vi "Astar on Occupancy Grid.vi"() -> ()   [LabVIEW 2017]
doc: "This example shows how to use the A* algorithm with an occupancy grid to compute the shortest path between start and goal nodes."
uses:
  <vilib>/robotics/Navigation/shared/WorldMap/OccupancyGridWorldMap/NI_Robotics_OccupancyGridWorldMap.lvclass
panel:
  in  "Save Grid":bool
  in  "Load Grid":bool
  in  "Action":enum32{"Mark Obstacle", "Set Start", "Set Goal"}(radio)
  in  "stop":bool
  out "Intensity Graph":dbl[][](graph)
  # "This example uses the A* algorithm to compute the shortest path between a start node and a goal node on an occupancy grid.\n\n1. Click the grid with Mark Obstacle selected to add or remove obstacles in the occupancy grid.\n\n2. Click the grid with Set Start or Set Goal selected to move the start and goal nodes of the shortest path.\n\n3. Click the Save button to save the current occupancy grid to a tab delimited text file.\n\n4. Click the Load button to load an occupancy grid from a tab delimited text file."
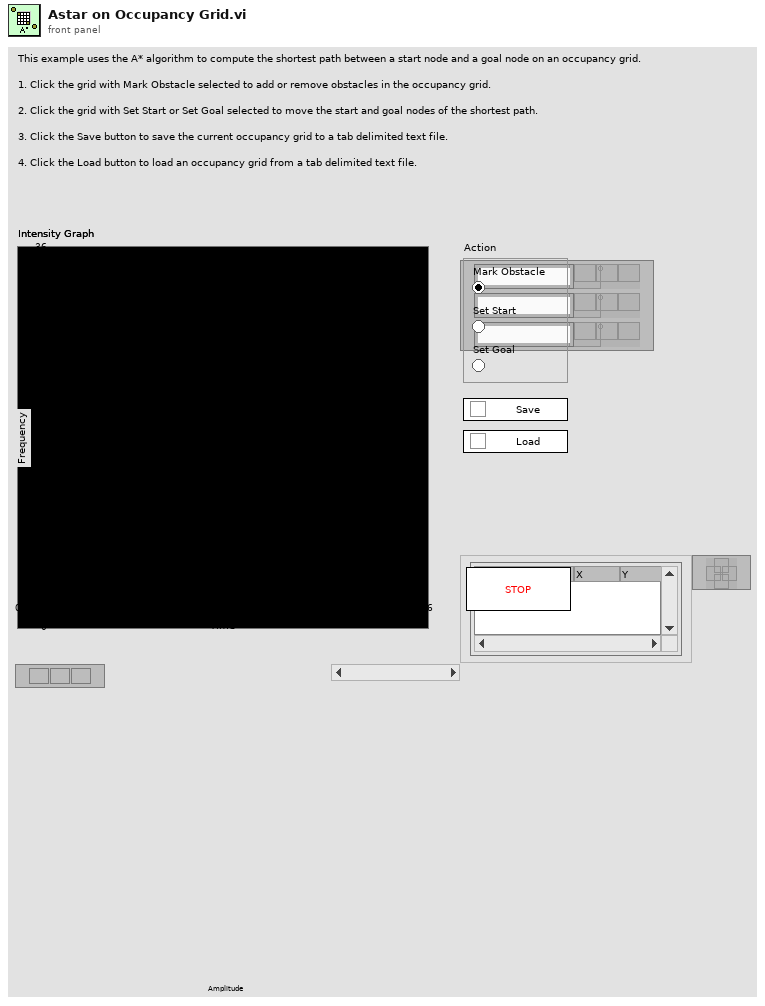
[diagram p1: front panel]
types:
  T1 = typedef "LVPoint32TypeDef.ctl" = cluster{"Horizontal":i32, "Vertical":i32}
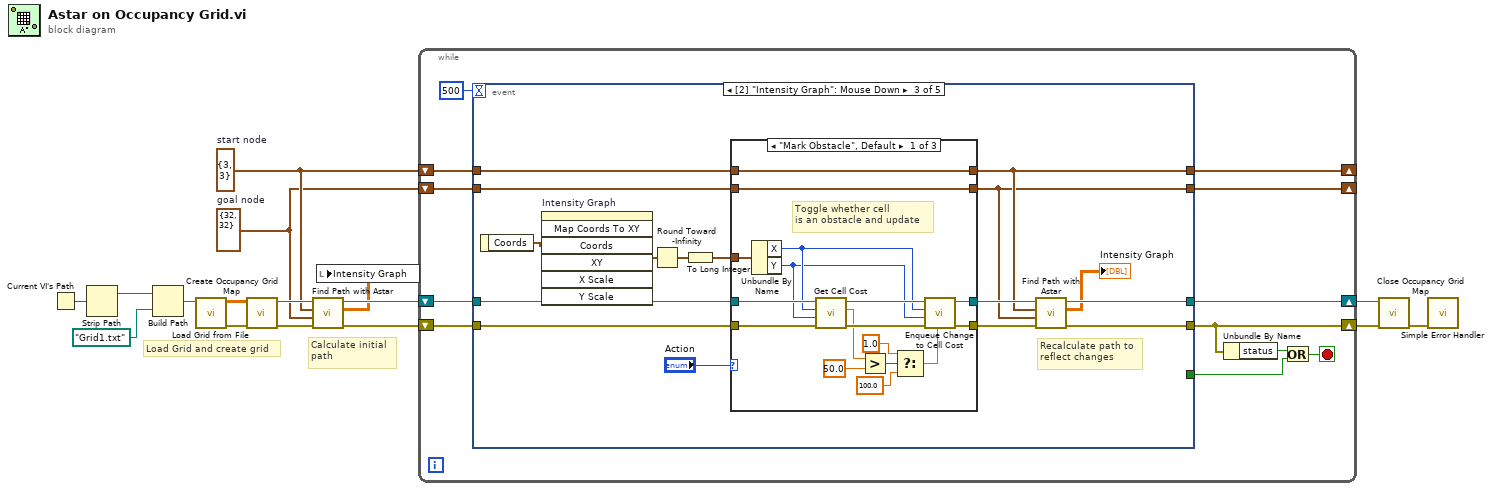
[diagram p0: block diagram]
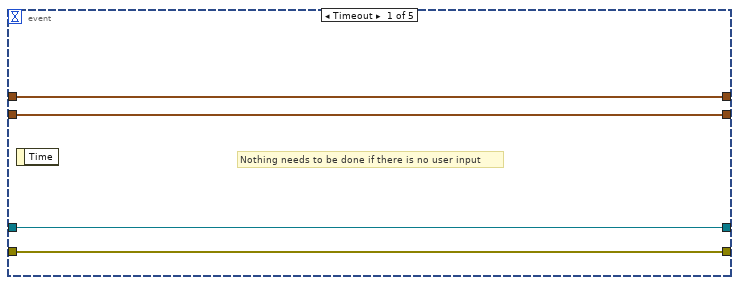
[diagram p2: hidden frame]
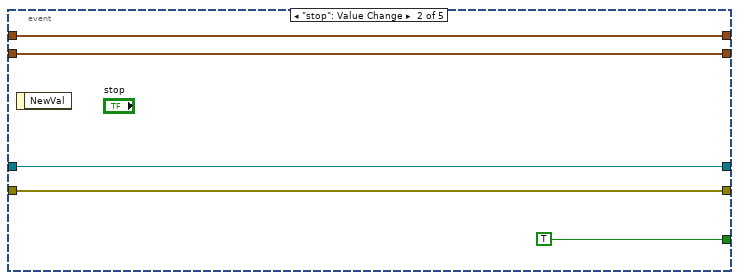
[diagram p3: hidden frame]
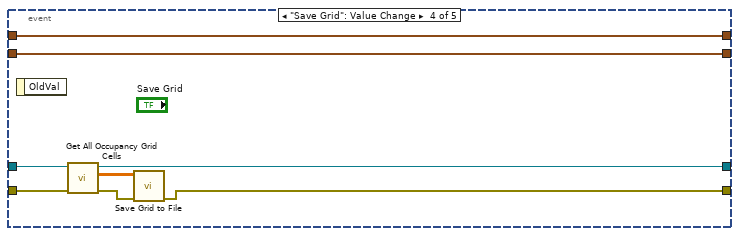
[diagram p6: hidden frame]
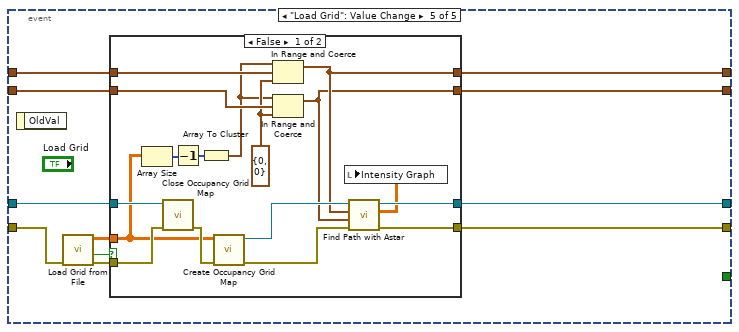
[diagram p7: hidden frame]
diagram:
  w2 = cluster{"X":i32, "Y":i32} {"X"=32, "Y"=32}  # goal node
  w3 = cluster{"X":i32, "Y":i32} {"X"=3, "Y"=3}  # start node
  # "Calculate initial \npath"
  # "Load Grid and create grid"
  n1 = Current VI's Path() -> (path=w14:path)
  n2 = Strip Path(path=w14) -> (stripped path=w13:path)  [unwired: 1 out]
  n3 = Build Path(base path=w13, name or relative path=path "Grid1.txt" ("stripped path")) -> (appended path=w11:path)
  n4 = call "Load Grid from File.vi"("file path"=w11) -> ("error out"=w9:errorcluster, "occupancy grid"=w10:dbl[][])  [unwired: 8 in, 1 out]
  n5 = call <vilib>:"Create Occupancy Grid Map.vi"("error in (no error)"=w9, "occupancy grid"=w10) -> ("error out"=w5:errorcluster, "map reference out"=w7:refnum<data-value>)  [unwired: 8 in]
  n6 = call "Find Path with Astar.vi"("error in (no error)"=w5, "goal node"=w2, "start node"=w3, "map reference in"=w7) -> ("error out"=w4:errorcluster, "intensity values"=w1:dbl[][], "map reference out"=w6:refnum<data-value>)  [unwired: 5 in]
  n7 = local write "Intensity Graph"(w1) -> ()
  n8 = while {
    shift-right: [w23] -> w16
    shift-left: w4 -> [w24]
    shift-right: [w19] -> _
    shift-left: w3 -> [w21]
    shift-right: [w18] -> _
    shift-left: w2 -> [w20]
    shift-right: [w17] -> w8
    shift-left: w6 -> [w25]
    stop <- w26 stop-if-true
    n9 = event shown="[2] \"Intensity Graph\": Mouse Down" {
      selector: _ -> [_ _ _ _ _]
      dyn-events: _ -> [_ _ _ _ _]
      timeout: 500 -> [_ _ _ _ _]
      tunnel: [_ TRUE _ _ _] -> w27
      tunnel: w25 -> [w31 w35 w50 w85 w95]
      tunnel: w24 -> [w32 w36 w49 w86 w97]
      tunnel: [w32 w36 w39 w82 w92] -> w23
      tunnel: [w31 w35 w40 w83 w91] -> w17
      tunnel: w21 -> [w30 w34 w47 w80 w90]
      tunnel: w20 -> [w29 w33 w46 w79 w89]
      tunnel: [w30 w34 w42 w80 w88] -> w19
      tunnel: [w29 w33 w41 w79 w87] -> w18
      event Timeout {
        # "Nothing needs to be done if there is no user input"
        n10 = event-data() -> ()  [unwired: 1 in, 1 out]
      }
      event "stop": Value Change {
        n11 = event-data() -> ()  [unwired: 1 in, 1 out]
      }
      event "Intensity Graph": Mouse Down {
        # "Recalculate path to\nreflect changes"
        n12 = event-data() -> ("Coords"=w53:T1)  [unwired: 1 in]
        n13 = invoke on="Intensity Graph" class="IntGraph (strict)" method="Map Coords To XY"("Coords"=w53) -> ("XY"=w52:cluster{"X":dbl, "Y":dbl})  [unwired: 6 in, 6 out]
        n14 = Round Toward -Infinity(1:w52) -> (0:w51:cluster{"X":dbl, "Y":dbl})
        n15 = To Long Integer(number=w51) -> (32bit integer=w45:cluster{"X":i32, "Y":i32})
        n16 = case shown="\"Mark Obstacle\", Default" "Action" {
          tunnel: w50 -> [w70 w72 w76]
          tunnel: w49 -> [w68 w71 w75]
          tunnel: [w60 w71 w75] -> w43
          tunnel: [w59 w72 w76] -> w44
          tunnel: w47 -> [w58 _ w78]
          tunnel: w46 -> [w57 w74 _]
          tunnel: [w58 w73 w78] -> w42
          tunnel: [w57 w74 w77] -> w41
          tunnel: w45 -> [w54 w73 w77]
          frame "Mark Obstacle", Default {
            # "Toggle whether cell\nis an obstacle and update"
            n17 = Unbundle By Name(w54) -> ("X"=w56:i32, "Y"=w55:i32)
            n18 = call <vilib>:"Get Cell Cost.vi"("error in (no error)"=w68, "y"=w55, "x"=w56, "map reference in"=w70) -> ("error out"=w67:errorcluster, "cost"=w66:dbl, "map reference out"=w69:refnum<data-value>)  [unwired: 4 in, 1 out]
            n19 = Greater?(x=w66, y=50.0) -> (0:w64:bool)
            n20 = Select(t=1.0, s=w64, f=100.0) -> (s? t:f=w61:dbl)
            n21 = call <vilib>:"Enqueue Change to Cell Cost.vi"("cost"=w61, "error in (no error)"=w67, "y"=w55, "x"=w56, "map reference in"=w69) -> ("error out"=w60:errorcluster, "map reference out"=w59:refnum<data-value>)  [unwired: 5 in]
          }
          frame "Set Start" {
            # "Change start node"
          }
          frame "Set Goal" {
            # "change goal node"
          }
        }
        n22 = call "Find Path with Astar.vi"("error in (no error)"=w43, "goal node"=w41, "start node"=w42, "map reference in"=w44) -> ("error out"=w39:errorcluster, "intensity values"=→"Intensity Graph":dbl[][], "map reference out"=w40:refnum<data-value>)  [unwired: 5 in]
      }
      event "Save Grid": Value Change {
        n23 = event-data() -> ()  [unwired: 1 in, 1 out]
        n24 = call <vilib>:"Get All Occupancy Grid Cells.vi"("error in (no error)"=w86, "map reference in"=w85) -> ("error out"=w84:errorcluster, "occupancy grid"=w81:dbl[][], "map reference out"=w83:refnum<data-value>)  [unwired: 7 in]
        n25 = call "Save Grid to File.vi"("error in (no error)"=w84, "occupancy grid"=w81) -> ("error out"=w82:errorcluster)  [unwired: 9 in]
      }
      event "Load Grid": Value Change {
        n26 = event-data() -> ()  [unwired: 1 in, 1 out]
        n27 = call "Load Grid from File.vi"("error in (no error)"=w97) -> ("error out"=w94:errorcluster, "cancelled"=w96:bool, "occupancy grid"=w93:dbl[][])  [unwired: 8 in]
        n28 = case shown="False" w96 {
          tunnel: w95 -> [w114 w118]
          tunnel: w94 -> [w113 w117]
          tunnel: w93 -> [w109 _]
          tunnel: [w104 w118] -> w91
          tunnel: [w100 w117] -> w92
          tunnel: w90 -> [w111 w116]
          tunnel: w89 -> [w110 w115]
          tunnel: [w103 w116] -> w88
          tunnel: [w102 w115] -> w87
          frame False {
            w108 = cluster{"X":i32, "Y":i32} {"X"=0, "Y"=0} ("lower limit")
            n29 = Array Size(array=w109) -> (size(s)=w107:i32[])
            n30 = call <vilib>:"Close Occupancy Grid Map.vi"("error in (no error)"=w113, "map reference in"=w114) -> ("error out"=w112:errorcluster)  [unwired: 9 in]
            n31 = Decrement(x=w107) -> (x-1=w98:i32[])
            n32 = Array To Cluster(array=w98) -> (cluster=w106:cluster{"[0]":i32, "[1]":i32})
            n33 = call <vilib>:"Create Occupancy Grid Map.vi"("error in (no error)"=w112, "occupancy grid"=w109) -> ("error out"=w101:errorcluster, "map reference out"=w105:refnum<data-value>)  [unwired: 8 in]
            n34 = In Range and Coerce(upper limit=w106, x=w111, lower limit=w108) -> (coerced(x)=w103:cluster{"[0]":i32, "[1]":i32})  [unwired: 1 out]
            n35 = In Range and Coerce(upper limit=w106, x=w110, lower limit=w108) -> (coerced(x)=w102:cluster{"[0]":i32, "[1]":i32})  [unwired: 1 out]
            n36 = call "Find Path with Astar.vi"("error in (no error)"=w101, "goal node"=w102, "start node"=w103, "map reference in"=w105) -> ("error out"=w100:errorcluster, "intensity values"=w99:dbl[][], "map reference out"=w104:refnum<data-value>)  [unwired: 5 in]
            n37 = local write "Intensity Graph"(w99) -> ()
          }
          frame True {
          }
        }
      }
    }
    n38 = Unbundle By Name(w23) -> ("status"=w22:bool)
    n39 = Or(x=w22, y=w27) -> (x .or. y?=w26:bool)
  }
  n40 = call <vilib>:"Close Occupancy Grid Map.vi"("error in (no error)"=w16, "map reference in"=w8) -> ("error out"=w15:errorcluster)  [unwired: 9 in]
  n41 = call <vilib>:"Simple Error Handler.vi"("error in (no error)"=w15) -> ()  [unwired: 4 in, 5 out]
